vi "Write Target.vi"(6 "amps?":bool caption="Amps", 7 "target":dbl caption="Target") -> (1 "unit":string caption="Unit", 2 "targetOUT":dbl caption="Target", 3 "display":string caption="Display")   [LabVIEW 2009, in "Magnet.lvclass"]
uses:
  Magnet.lvclass
  Global/Power Supply.vi
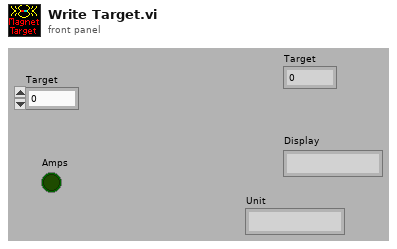
[diagram p1: front panel]
types:
  T1 = typedef "PSIO.ctl" = cluster{"Address":T2, "Version":enum16{"PS", "IPS"}}
  T2 = typedef "OxfordAddress.ctl" = cluster{"Com Port":i32, "ISOBUS Address":i32, "GPIB Address":i16, "Communication":enum16{"RS232", "ISOBUS", "GPIB", "Gateway"}}
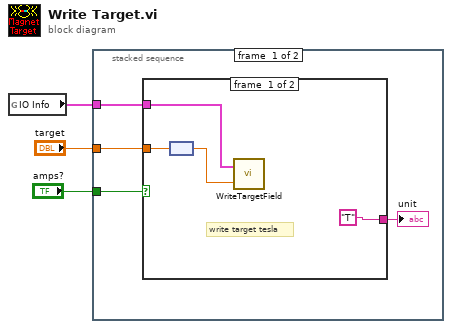
[diagram p0: block diagram]
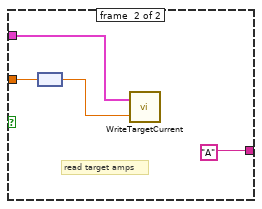
[diagram p2: hidden frame]
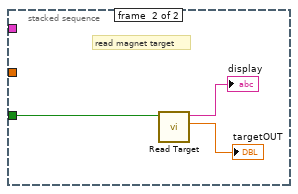
[diagram p3: hidden frame]
diagram:
  n1 = global read "Power Supply.vi" "IO Info"() -> (w1:T1)
  n2 = stacked-sequence {
    tunnel: "amps?" -> [w7 w18]
    tunnel: "target" -> [w6 _]
    tunnel: w1 -> [w5 _]
    frame #0 {
      n3 = case shown="False" w7 {
        tunnel: w6 -> [w11 w15]
        tunnel: w5 -> [w9 w13]
        tunnel: ["T" "A"] -> w4
        frame #0 {
          # "write target tesla"
          n4 = node(w11) -> (w10:dbl[unit])
          n5 = call "WriteTargetField.vi"("Target Field"=w10, "IO Info"=w9) -> ()  [unwired: 2 out]
        }
        frame #1 {
          # "read target amps"
          n6 = node(w15) -> (w14:dbl[unit])
          n7 = call "WriteTargetCurrent.vi"("Current"=w14, "IO Info"=w13) -> ()  [unwired: 2 out]
        }
      }
      "unit" <- w4
    }
    frame #1 {
      # "read magnet target"
      n8 = call "Read Target.vi"("amps?"=w18) -> ("target"=→"targetOUT":dbl, "display"=→"display":string)  [unwired: 5 out]
    }
  }
